vi "01_Serial_Response.vi"(4 "Read":string) -> (1 "Response":string)   [LabVIEW 2020]
panel:
  in  "LWST":i16
  in  "Persist":bool caption="Persistent Error?"
  in  "OBS OFF":bool
  in  "OBS ON":bool
  out "STEPS TIMER":u32
  out "STEP":u8
  out "LED2":u16 format="%.0x"
  in  "EDGA":i16
  out "SPM":u8
  in  "ERR":u8
  in  "RES BAD":bool
  in  "RAMP BAD":bool
  in  "LOOP":u16=19543
  in  "MAMP":u16
  in  "VBUS":u16=153
  in  "LFTG":u16
  in  "LFTS":u16
  in  "LIFT":u16=1256
  in  "BRK":u16
  in  "PRPM":u16
  in  "RPM":u16
  in  "ACAD":u16=1
  in  "BATL":u16
  in  "BATC":u16=1
  in  "VCHG":u16=130
  in  "VBAT":u16=130
  in  "TYPE":u16=32
  in  "VER":u16=951
  in  "ASL Part Num":string="304029-101 007"
  out "EERD":string[](array[string])
  out "SECS TIMER":u32
  in  "SECS VALUE":u8=255
  in  "Simulate Stop":bool
  in  "Minor Part Num":string="305531-101 909"
  out "REV":u8
  out "Array":string[](array[string])
  in  "Lower Part Num":string="305530-101 951"
  in  "Delay":u64
  # "Configured for SCL800"
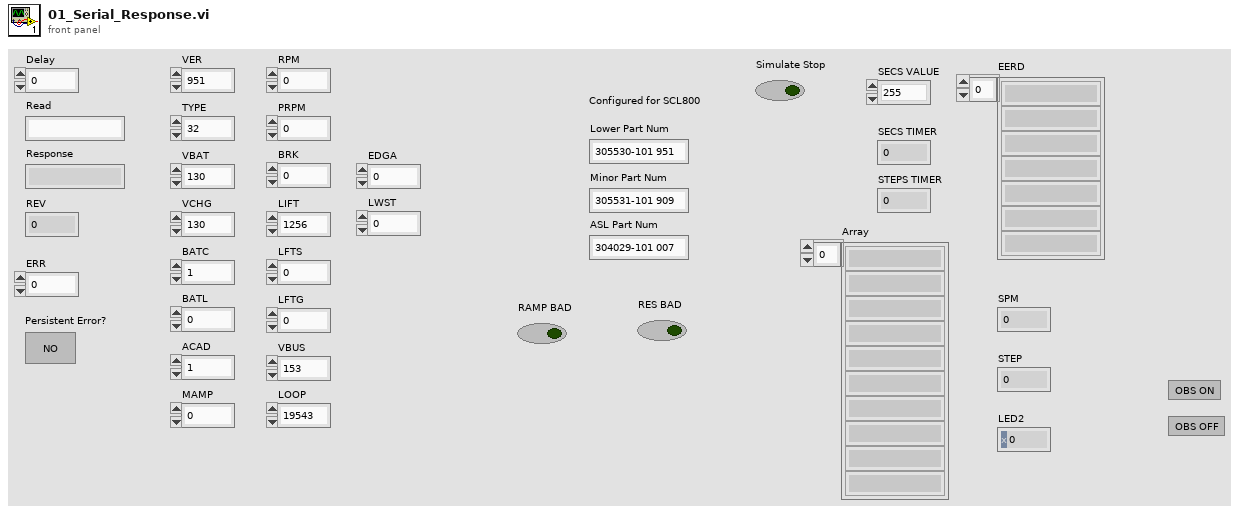
[diagram p1: front panel]
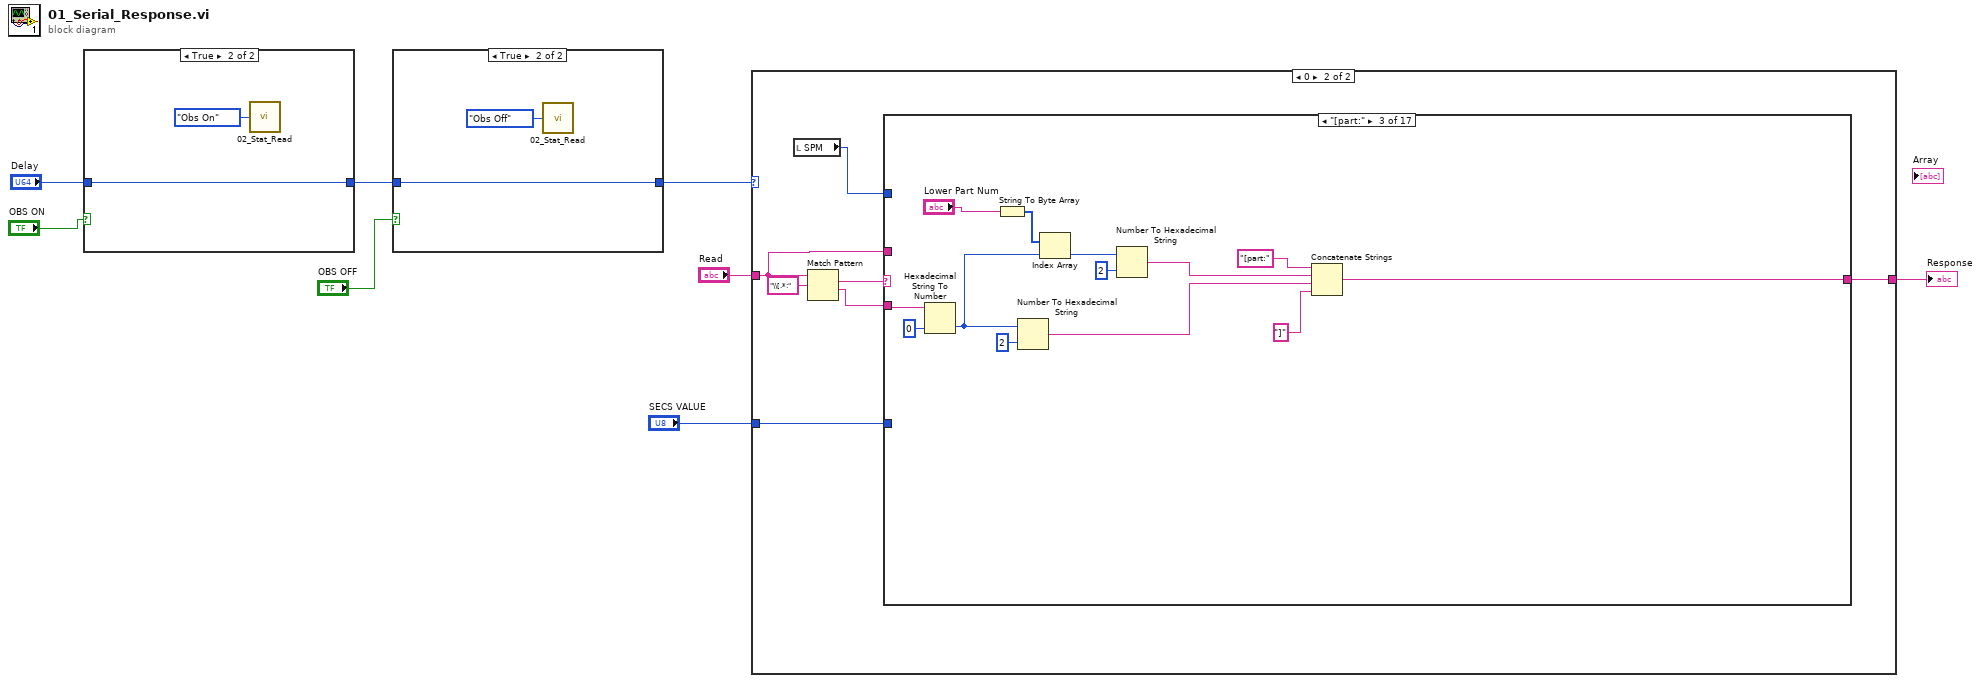
[diagram p0: block diagram]
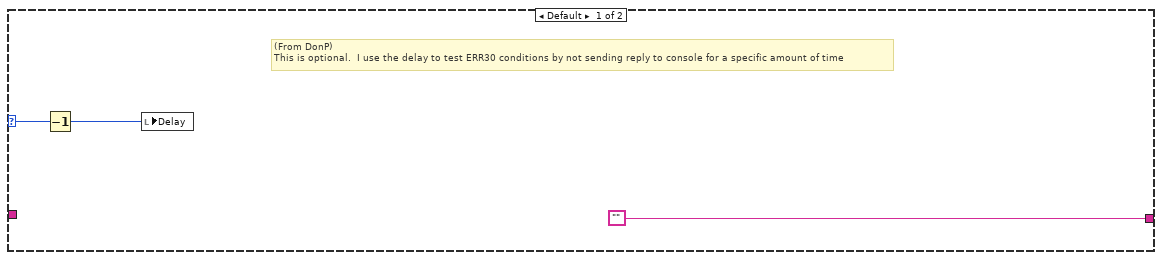
[diagram p4: hidden frame]
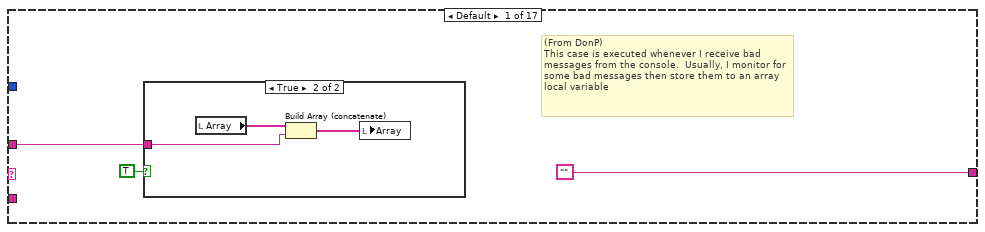
[diagram p5: hidden frame]
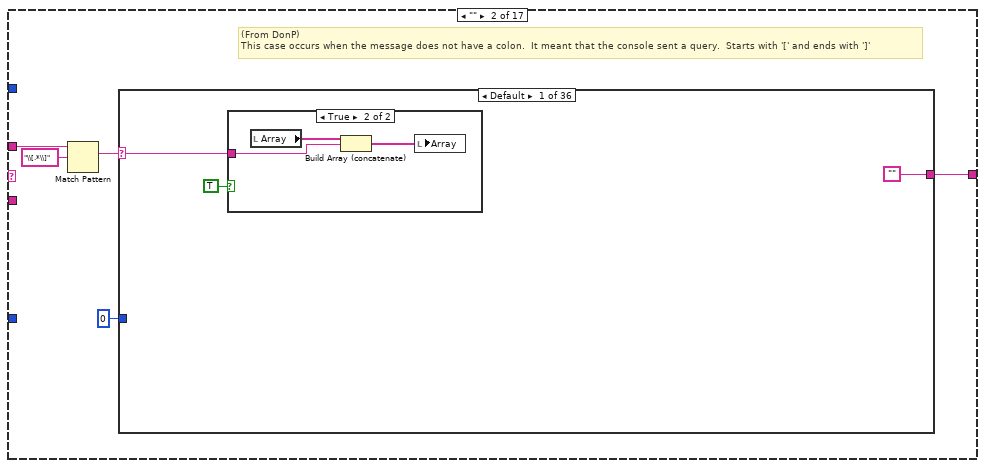
[diagram p7: hidden frame]
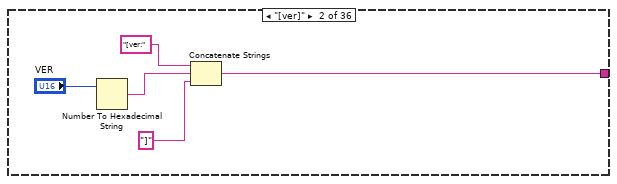
[diagram p9: hidden frame]
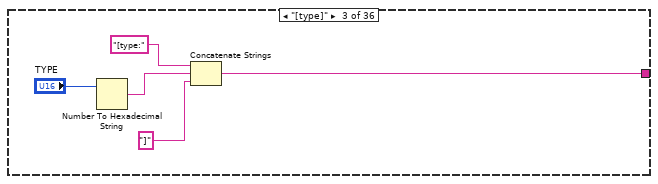
[diagram p10: hidden frame]
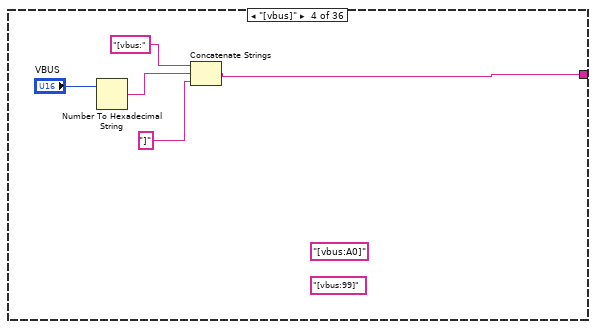
[diagram p11: hidden frame]
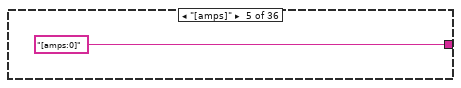
[diagram p12: hidden frame]
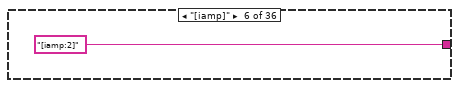
[diagram p13: hidden frame]
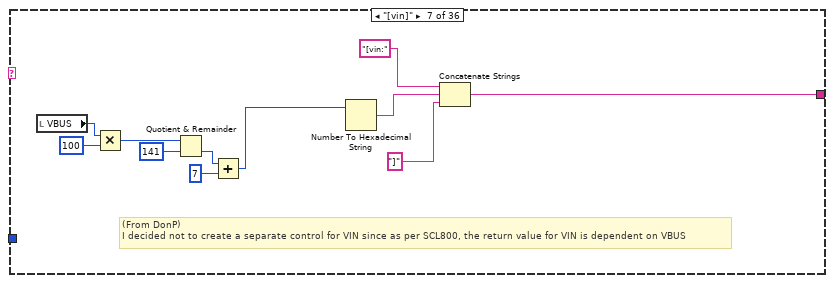
[diagram p14: hidden frame]
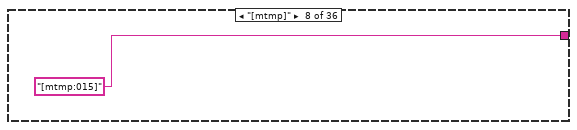
[diagram p15: hidden frame]
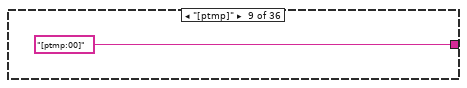
[diagram p16: hidden frame]
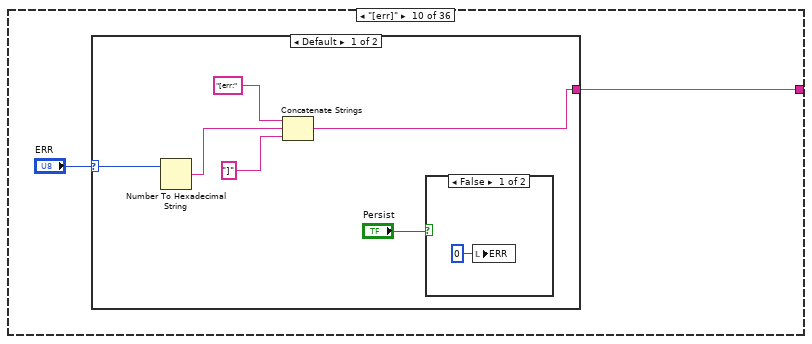
[diagram p17: hidden frame]
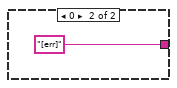
[diagram p19: hidden frame]
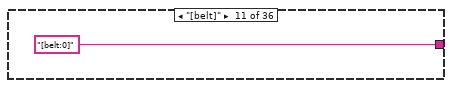
[diagram p20: hidden frame]
diagram:
  n1 = case shown="True" "OBS ON" {
    tunnel: "Delay" -> [w9 w11]
    tunnel: [w9 w11] -> w5
    frame False {
    }
    frame True {
      n2 = call "02_Stat_Read.vi"("Command"=enum16{"Init", "Read", "Obs On", "Obs Off"}."Obs On") -> ()  [unwired: 1 out]
    }
  }
  n3 = case shown="True" "OBS OFF" {
    tunnel: w5 -> [w12 w14]
    tunnel: [w12 w14] -> w4
    frame False {
    }
    frame True {
      n4 = call "02_Stat_Read.vi"("Command"=enum16{"Init", "Read", "Obs On", "Obs Off"}."Obs Off") -> ()  [unwired: 1 out]
    }
  }
  n5 = case shown="0" w4 {
    selector: w4 -> [w16 _]
    tunnel: "Read" -> [_ w19]
    tunnel: ["" w22] -> w7
    tunnel: "SECS VALUE" -> [_ w20]
    frame Default {
      # "(From DonP)\nThis is optional.  I use the delay to test ERR30 conditions by not sending reply to console for a specific amount of time"
      n6 = Decrement(x=w16) -> (x-1=w15:u64)
      n7 = local write "Delay"(w15) -> ()
    }
    frame 0 {
      n8 = local read "SPM"() -> (w18:u8)
      n9 = Match Pattern(string=w19, regular expression="\\[.*:") -> (match substring=w23:string, after substring=w21:string)  [unwired: 1 in, 2 out]
      n10 = case shown="\"[part:\"" w23 {
        tunnel: ["" w33 w234 w247 w260 w271 w278 w294 w305 w311 w324 "[rmpd:AA]" ("Response") "[clr:0]" ("Response") w349 w360 w365 w373] -> w22
        tunnel: w21 -> [_ _ w244 w257 w270 w277 w284 w299 w310 w312 w329 w334 w342 w353 w364 w367 w374]
        tunnel: w20 -> [_ _ _ _ _ _ _ _ _ _ _ _ _ _ _ _ _]
        tunnel: w19 -> [w26 w31 _ _ _ _ _ _ _ _ _ _ _ _ _ _ _]
        tunnel: w18 -> [_ _ _ _ _ _ _ w293 _ _ _ _ _ _ _ _ _]
        frame Default {
          # "(From DonP)\nThis case is executed whenever I receive bad messages from the console.  Usually, I monitor for some bad messages then store them to an array local variable"
          n11 = case shown="True" TRUE {
            tunnel: w26 -> [_ w28]
            frame False {
            }
            frame True {
              n12 = local read "Array"() -> (w30:string[])
              n13 = Build Array (concatenate)(w30, w28) -> (w29:string[])
              n14 = local write "Array"(w29) -> ()
            }
          }
        }
        frame "" {
          # "(From DonP)\nThis case occurs when the message does not have a colon.  It meant that the console sent a query.  Starts with '[' and ends with ']'"
          n15 = Match Pattern(string=w31, regular expression="\\[.*\\]") -> (match substring=w34:string)  [unwired: 1 in, 3 out]
          n16 = case shown="Default" w34 {
            selector: w34 -> [w37 _ _ _ _ _ _ _ _ _ _ _ _ _ _ _ _ _ _ _ _ _ _ _ _ _ _ _ _ _ _ _ _ _ _ _]
            tunnel: ["" w42 w47 w52 "[amps:0]" "[iamp:2]" w66 "[mtmp:015]" "[ptmp:00]" w72 "[belt:0]" w83 w88 w93 "[inc]" w99 w104 w109 w114 w119 w128 w142 w149 w159 "[rpml:0]" "[rpmh:39]" w166 "[bld:1D]" "[stop]" w173 w180 w187 w208 w216 w223 w227] -> w33
            tunnel: u8 0 ("SECS VALUE") -> [_ _ _ _ _ _ _ _ _ _ _ _ _ _ _ _ _ _ _ _ w130 _ w147 _ _ _ _ _ _ _ _ _ _ _ _ _]
            frame Default {
              n17 = case shown="True" TRUE {
                tunnel: w37 -> [_ w39]
                frame False {
                }
                frame True {
                  n18 = local read "Array"() -> (w41:string[])
                  n19 = Build Array (concatenate)(w41, w39) -> (w40:string[])
                  n20 = local write "Array"(w40) -> ()
                }
              }
            }
            frame "[ver]" {
              n21 = Number To Hexadecimal String(2:"VER") -> (0:w44:string)  [unwired: 1 in]
              n22 = Concatenate Strings("[ver:", w44, "]") -> (w42:string)
            }
            frame "[type]" {
              n23 = Number To Hexadecimal String(2:"TYPE") -> (0:w49:string)  [unwired: 1 in]
              n24 = Concatenate Strings("[type:", w49, "]") -> (w47:string)
            }
            frame "[vbus]" {
              (unwired) "[vbus:99]"
              (unwired) "[vbus:A0]"
              n25 = Number To Hexadecimal String(2:"VBUS") -> (0:w54:string)  [unwired: 1 in]
              n26 = Concatenate Strings("[vbus:", w54, "]") -> (w52:string)
            }
            frame "[amps]" {
            }
            frame "[iamp]" {
            }
            frame "[vin]" {
              # "(From DonP)\nI decided not to create a separate control for VIN since as per SCL800, the return value for VIN is dependent on VBUS"
              n27 = local read "VBUS"() -> (w65:u16)
              n28 = Multiply(x=w65, y=u16 100) -> (x*y=w63:u16)
              n29 = Quotient & Remainder(x=w63, y=u16 141) -> (floor(x/y)=w61:u16)  [unwired: 1 out]
              n30 = Add(x=w61, y=u16 7) -> (x+y=w59:u16)
              n31 = Number To Hexadecimal String(2:w59) -> (0:w69:string)  [unwired: 1 in]
              n32 = Concatenate Strings("[vin:", w69, "]") -> (w66:string)
            }
            frame "[mtmp]" {
            }
            frame "[ptmp]" {
            }
            frame "[err]" {
              n33 = case shown="Default" "ERR" {
                selector: "ERR" -> [w79 _]
                tunnel: [w75 "[err]"] -> w72
                frame Default {
                  n34 = Number To Hexadecimal String(2:w79) -> (0:w78:string)  [unwired: 1 in]
                  n35 = Concatenate Strings("[err:" ("string"), w78, "]" ("string")) -> (w75:string)
                  n36 = case shown="False" "Persist" {
                    frame False {
                      n37 = local write "ERR"(u8 0 ("ERR")) -> ()
                    }
                    frame True {
                    }
                  }
                }
                frame 0 {
                }
              }
            }
            frame "[belt]" {
            }
            frame "[lift]" {
              n38 = Number To Hexadecimal String(2:"LIFT") -> (0:w85:string)  [unwired: 1 in]
              n39 = Concatenate Strings("[lift:", w85, "]") -> (w83:string)
            }
            frame "[lfts]" {
              n40 = Number To Hexadecimal String(2:"LFTS") -> (0:w90:string)  [unwired: 1 in]
              n41 = Concatenate Strings("[lfts:", w90, "]") -> (w88:string)
            }
            frame "[lftg]" {
              n42 = Number To Hexadecimal String(2:"LFTG") -> (0:w95:string)  [unwired: 1 in]
              n43 = Concatenate Strings("[lftg:", w95, "]") -> (w93:string)
            }
            frame "[inc]" {
            }
            frame "[vbat]" {
              n44 = Number To Hexadecimal String(2:"VBAT") -> (0:w101:string)  [unwired: 1 in]
              n45 = Concatenate Strings("[vbat:", w101, "]") -> (w99:string)
            }
            frame "[vchg]" {
              n46 = Number To Hexadecimal String(2:"VCHG") -> (0:w106:string)  [unwired: 1 in]
              n47 = Concatenate Strings("[vchg:", w106, "]") -> (w104:string)
            }
            frame "[batc]" {
              n48 = Number To Hexadecimal String(2:"BATC") -> (0:w111:string)  [unwired: 1 in]
              n49 = Concatenate Strings("[batc:", w111, "]") -> (w109:string)
            }
            frame "[batl]" {
              n50 = Number To Hexadecimal String(2:"BATL") -> (0:w116:string)  [unwired: 1 in]
              n51 = Concatenate Strings("[batl:", w116, "]") -> (w114:string)
            }
            frame "[acad]" {
              n52 = Number To Hexadecimal String(2:"ACAD") -> (0:w121:string)  [unwired: 1 in]
              n53 = Concatenate Strings("[acad:", w121, "]") -> (w119:string)
            }
            frame "[secs]" {
              n54 = case shown="True" "Simulate Stop" {
                tunnel: w130 -> [_ _]
                tunnel: [u8 255 ("SECS VALUE") w135] -> w124
                tunnel: [w132 w136] -> w125
                frame False {
                  n55 = Tick Count (ms)() -> (millisecond timer value=w132:u32)
                }
                frame True {
                  n56 = local read "SECS TIMER"() -> (w136:u32)
                  n57 = Tick Count (ms)() -> (millisecond timer value=w139:u32)
                  n58 = Add(x=w136, y=u32 60000) -> (x+y=w140:u32)
                  n59 = Subtract(x=w140, y=w139) -> (x-y=w138:u32)
                  n60 = Quotient & Remainder(x=w138, y=u32 1000) -> (floor(x/y)=w134:u32)  [unwired: 1 out]
                  n61 = To Unsigned Byte Integer(number=w134) -> (unsigned 8bit integer=w135:u8)
                }
              }
              "SECS TIMER" <- w125
              n62 = Number To Hexadecimal String(2:w124) -> (0:w126:string)  [unwired: 1 in]
              n63 = local write "SECS VALUE"(w124) -> ()
              n64 = Concatenate Strings("[secs:" ("string"), w126, "]" ("string")) -> (w128:string)
            }
            frame "[rpm]" {
              n65 = Number To Hexadecimal String(2:"RPM") -> (0:w144:string)  [unwired: 1 in]
              n66 = Concatenate Strings("[rpm:", w144, "]") -> (w142:string)
            }
            frame "[rev]" {
              n67 = case shown="Default" w147 {
                tunnel: [w154 w155] -> w148
                frame Default {
                  n68 = local read "REV"() -> (w154:u8)
                }
                frame 255 {
                  n69 = Tick Count (ms)() -> (millisecond timer value=w158:u32)
                  n70 = Quotient & Remainder(x=w158, y=u32 1000) -> (floor(x/y)=w156:u32)  [unwired: 1 out]
                  n71 = To Unsigned Byte Integer(number=w156) -> (unsigned 8bit integer=w155:u8)
                }
              }
              "REV" <- w148
              n72 = Number To Hexadecimal String(1:i16 2 ("width (-)"), 2:w148) -> (0:w153:string)
              n73 = Concatenate Strings("[rev:" ("string"), w153, "]" ("string")) -> (w149:string)
            }
            frame "[prpm]" {
              n74 = Number To Hexadecimal String(2:"PRPM") -> (0:w161:string)  [unwired: 1 in]
              n75 = Concatenate Strings("[prpm:", w161, "]") -> (w159:string)
            }
            frame "[rpml]" {
            }
            frame "[rpmh]" {
            }
            frame "[brk]" {
              n76 = Number To Hexadecimal String(2:"BRK") -> (0:w168:string)  [unwired: 1 in]
              n77 = Concatenate Strings("[brk:", w168, "]") -> (w166:string)
            }
            frame "[bld]" {
            }
            frame "[stop]" {
            }
            frame "[mamp]" {
              n78 = Number To Hexadecimal String(2:"MAMP") -> (0:w175:string)  [unwired: 1 in]
              n79 = Concatenate Strings("[mamp:", w175, "]") -> (w173:string)
            }
            frame "[stat]" {
              n80 = call "02_Stat_Read.vi"("Command"=enum16{"Init", "Read", "Obs On", "Obs Off"}."Read") -> ("STAT"=w179:u32)
              n81 = Number To Hexadecimal String(2:w179) -> (0:w182:string)  [unwired: 1 in]
              n82 = Concatenate Strings("[stat:", w182, "]") -> (w180:string)
            }
            frame "[step]" {
              n83 = local read "SPM"() -> (w186:u8)
              n84 = case shown="0" w186 {
                selector: w186 -> [w200 _]
                tunnel: [w192 w207] -> w185
                tunnel: [w193 w206] -> w184
                frame Default {
                  n85 = local read "STEPS TIMER"() -> (w194:u32)
                  n86 = Quotient & Remainder(x=u32 60000, y=w200) -> (floor(x/y)=w198:u32)  [unwired: 1 out]
                  n87 = Tick Count (ms)() -> (millisecond timer value=w197:u32)
                  n88 = Add(x=w198, y=w194) -> (x+y=w191:u32)
                  n89 = local read "STEP"() -> (w195:u8)
                  n90 = Greater?(x=w197, y=w191) -> (0:w196:bool)
                  n91 = case shown="True" w196 {
                    tunnel: w195 -> [w201 w205]
                    tunnel: w194 -> [w202 _]
                    tunnel: [w202 w203] -> w193
                    tunnel: [w201 w204] -> w192
                    tunnel: w191 -> [_ w203]
                    frame False {
                    }
                    frame True {
                      n92 = Increment(x=w205) -> (x+1=w204:u8)
                    }
                  }
                }
                frame 0 {
                  n93 = local read "STEP"() -> (w207:u8)
                  n94 = Tick Count (ms)() -> (millisecond timer value=w206:u32)
                }
              }
              "STEP" <- w185
              "STEPS TIMER" <- w184
              n95 = Number To Hexadecimal String(2:w185) -> (0:w189:string)  [unwired: 1 in]
              n96 = Concatenate Strings("[step:", w189, "]") -> (w187:string)
            }
            frame "[edga]" {
              n97 = Number To Hexadecimal String(2:"EDGA") -> (0:w210:string)  [unwired: 1 in]
              n98 = Concatenate Strings("[edga:", w210, "]") -> (w208:string)
            }
            frame "[spma]" {
              n99 = local read "SPM"() -> (w215:u8)
              n100 = Multiply(x=w215, y=u8 10) -> (x*y=w214:u8)
              n101 = Number To Hexadecimal String(2:w214) -> (0:w218:string)  [unwired: 1 in]
              n102 = Concatenate Strings("[spma:", w218, "]") -> (w216:string)
            }
            frame "[spmb]" {
              n103 = local read "SPM"() -> (w222:u8)
              n104 = Multiply(x=w222, y=u8 10) -> (x*y=w221:u8)
              n105 = Number To Hexadecimal String(2:w221) -> (0:w225:string)  [unwired: 1 in]
              n106 = Concatenate Strings("[spmb:", w225, "]") -> (w223:string)
            }
            frame "[lwst]" {
              n107 = Number To Hexadecimal String(2:"LWST") -> (0:w229:string)  [unwired: 1 in]
              n108 = Concatenate Strings("[lwst:", w229, "]") -> (w227:string)
            }
          }
        }
        frame "[part:" {
          n109 = Hexadecimal String To Number(string=w244, default (0uL)=u8 0 ("default (0 U32)")) -> (number=w233:u8)  [unwired: 1 in, 1 out]
          n110 = String To Byte Array(string="Lower Part Num") -> (unsigned byte array=w241:u8[])
          n111 = Number To Hexadecimal String(1:i16 2 ("width (-)"), 2:w233) -> (0:w237:string)
          n112 = Index Array(array=w241, index=w233) -> (element=w239:u8)
          n113 = Number To Hexadecimal String(1:i16 2 ("width (-)"), 2:w239) -> (0:w238:string)
          n114 = Concatenate Strings("[part:" ("string"), w238, w237, "]" ("string")) -> (w234:string)
        }
        frame "[prts:" {
          n115 = Hexadecimal String To Number(string=w257, default (0uL)=u8 0 ("default (0 U32)")) -> (number=w246:u8)  [unwired: 1 in, 1 out]
          n116 = String To Byte Array(string="Minor Part Num") -> (unsigned byte array=w254:u8[])
          n117 = Number To Hexadecimal String(1:i16 2 ("width (-)"), 2:w246) -> (0:w250:string)
          n118 = Index Array(array=w254, index=w246) -> (element=w252:u8)
          n119 = Number To Hexadecimal String(1:i16 2 ("width (-)"), 2:w252) -> (0:w251:string)
          n120 = Concatenate Strings("[prts:" ("string"), w251, w250, "]" ("string")) -> (w247:string)
        }
        frame "[prta:" {
          n121 = Hexadecimal String To Number(string=w270, default (0uL)=u8 0 ("default (0 U32)")) -> (number=w259:u8)  [unwired: 1 in, 1 out]
          n122 = String To Byte Array(string="ASL Part Num") -> (unsigned byte array=w267:u8[])
          n123 = Number To Hexadecimal String(1:i16 2 ("width (-)"), 2:w259) -> (0:w263:string)
          n124 = Index Array(array=w267, index=w259) -> (element=w265:u8)
          n125 = Number To Hexadecimal String(1:i16 2 ("width (-)"), 2:w265) -> (0:w264:string)
          n126 = Concatenate Strings("[prta:" ("string"), w264, w263, "]" ("string")) -> (w260:string)
        }
        frame "[inc:" {
          (unwired) "[ESTOP:BAD]" ("t")
          n127 = Hexadecimal String To Number(string=w277, default (0uL)=u8 0 ("default (0 U32)")) -> (number=w272:u8)  [unwired: 1 in, 1 out]
          n128 = Number To Hexadecimal String(2:w272) -> (0:w275:string)  [unwired: 1 in]
          n129 = Concatenate Strings("[inc:" ("string"), w275, "]" ("string")) -> (w271:string)
        }
        frame "[mph:" {
          (unwired) "[ESTOP:BAD]" ("t")
          n130 = Hexadecimal String To Number(string=w284, default (0uL)=u8 0 ("default (0 U32)")) -> (number=w279:u8)  [unwired: 1 in, 1 out]
          n131 = case shown="Default" w279 {
            selector: w279 -> [_ w287]
            tunnel: ["0" w288] -> w282
            frame 0 {
            }
            frame Default {
              n132 = Decrement(x=w287) -> (x-1=w286:u8)
              n133 = Number To Hexadecimal String(2:w286) -> (0:w288:string)  [unwired: 1 in]
            }
          }
          n134 = Concatenate Strings("[mph:" ("string"), w282, "]" ("string")) -> (w278:string)
        }
        frame "[spm:" {
          n135 = Hexadecimal String To Number(string=w299, default (0uL)=u8 0 ("default (0 U32)")) -> (number=w292:u8)  [unwired: 1 in, 1 out]
          "SPM" <- w292
          n136 = Equal To 0?(x=w293) -> (x = 0?=w291:bool)
          n137 = Equal To 0?(x=w292) -> (x = 0?=w289:bool)
          n138 = Exclusive Or(1:w289, 2:w291) -> (0:w290:bool)
          n139 = Number To Hexadecimal String(2:w292) -> (0:w297:string)  [unwired: 1 in]
          n140 = case shown="True" w290 {
            tunnel: w289 -> [_ w303]
            frame False {
            }
            frame True {
              n141 = Select(t=i16 0 ("LWST"), s=w303, f=i16 3) -> (s? t:f=w300:i16)
              n142 = local write "LWST"(w300) -> ()
            }
          }
          n143 = Concatenate Strings("[spm:" ("string"), w297, "]" ("string")) -> (w294:string)
        }
        frame "[cnfg:" {
          n144 = Hexadecimal String To Number(string=w310, default (0uL)=u8 0 ("default (0 U32)")) -> (number=w304:u8)  [unwired: 1 in, 1 out]
          n145 = Number To Hexadecimal String(2:w304) -> (0:w308:string)  [unwired: 1 in]
          n146 = Concatenate Strings("[cnfg:" ("string"), w308, "]" ("string")) -> (w305:string)
        }
        frame "[loop:" {
          n147 = case shown="\"5550]\"" w312 {
            selector: w312 -> [w313 _]
            tunnel: ["" w317] -> w311
            frame Default {
              n148 = local read "Array"() -> (w315:string[])
              n149 = Build Array (concatenate)(w315, w313) -> (w314:string[])
              n150 = local write "Array"(w314) -> ()
            }
            frame "5550]" {
              n151 = Number To Hexadecimal String(2:"LOOP") -> (0:w319:string)  [unwired: 1 in]
              n152 = Concatenate Strings("[loop:", w319, "]") -> (w317:string)
            }
          }
        }
        frame "[led1:" {
          n153 = Hexadecimal String To Number(string=w329, default (0uL)=u8 0 ("default (0 U32)")) -> (number=w323:u8)  [unwired: 1 in, 1 out]
          n154 = Number To Hexadecimal String(1:i16 2 ("width (-)"), 2:w323) -> (0:w327:string)
          n155 = Concatenate Strings("[led1:" ("string"), w327, "]" ("string")) -> (w324:string)
        }
        frame "[rmpd:" {
          n156 = Hexadecimal String To Number(string=w334, default (0uL)=u8 0 ("default (0 U32)")) -> (number=w331:u8)  [unwired: 1 in, 1 out]
          n157 = Number To Hexadecimal String(1:i16 2 ("width (-)"), 2:w331) -> ()  [unwired: 1 out]
        }
        frame "[led2:" {
          n158 = Hexadecimal String To Number(string=w342, default (0uL)=u16 0 ("default (0 U32)")) -> (number=w335:u16)  [unwired: 1 in, 1 out]
          "LED2" <- w335
          n159 = Number To Hexadecimal String(1:i16 2 ("width (-)"), 2:w335) -> (0:w340:string)
          n160 = Concatenate Strings("[led2:" ("string"), w340, "]" ("string")) -> ()  [unwired: 1 out]
        }
        frame "[ramp:" {
          n161 = Hexadecimal String To Number(string=w353, default (0uL)=u8 0 ("default (0 U32)")) -> (number=w348:u8)  [unwired: 1 in, 1 out]
          n162 = Number To Hexadecimal String(1:i16 2 ("width (-)"), 2:w348) -> (0:w345:string)
          n163 = Select(t="BAD", s="RAMP BAD", f=w345) -> (s? t:f=w346:string)
          n164 = Concatenate Strings("[ramp:" ("string"), w346, "]" ("string")) -> (w349:string)
        }
        frame "[res:" {
          n165 = Hexadecimal String To Number(string=w364, default (0uL)=u8 0 ("default (0 U32)")) -> (number=w359:u8)  [unwired: 1 in, 1 out]
          n166 = Number To Hexadecimal String(1:i16 2 ("width (-)"), 2:w359) -> (0:w355:string)
          n167 = Select(t="BAD", s="RES BAD", f=w355) -> (s? t:f=w356:string)
          n168 = Concatenate Strings("[res:" ("string"), w356, "]" ("string")) -> (w360:string)
        }
        frame "[eerd:" {
          n169 = local read "EERD"() -> (w368:string[])
          n170 = Hexadecimal String To Number(string=w367) -> (number=w370:u32)  [unwired: 2 in, 1 out]
          n171 = call "01_AMT_EEROM.vi"("Number"=w370, "Command"=enum16{"Init", "EERD", "EEWR"}."EERD") -> ("Response"=w365:string)  [unwired: 1 in]
          n172 = Build Array (concatenate)(w368, w367) -> (→"EERD":string[])
        }
        frame "[eewr:" {
          n173 = Hexadecimal String To Number(string=w374) -> (number=w372:u32)  [unwired: 2 in, 1 out]
          n174 = call "01_AMT_EEROM.vi"("Number"=w372, "Command"=enum16{"Init", "EERD", "EEWR"}."EEWR") -> ("Response"=w373:string)  [unwired: 1 in]
        }
      }
    }
  }
  "Response" <- w7
